vi "Encoder Sim.vi"(2 "Direction":enum16{"A leads B, CCW", "B leads A, CW"}(ring), 3 "Period (s)":dbl=1.0 min=0.001 max=1.0 step=0.001) -> (0 "Actual Counts":i32, 1 "Encoder Signals":bool[](array[boolean]))   [LabVIEW 2017]
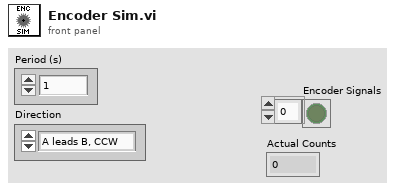
[diagram p1: front panel]
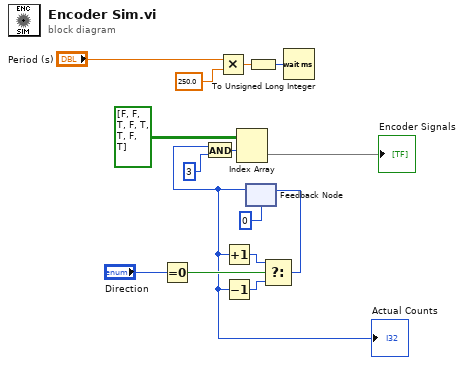
[diagram p0: block diagram]
diagram:
  n1 = Equal To 0?(x="Direction") -> (x = 0?=w8:bool)
  n2 = Multiply(x="Period (s)", y=250.0) -> (x*y=w6:dbl)
  n3 = feedback #1(0) -> (w1:i32)
  "Actual Counts" <- w1
  n4 = And(x=w1, y=3) -> (x .and. y?=w12:i32)
  n5 = Increment(x=w1) -> (x+1=w11:i32)
  n6 = Decrement(x=w1) -> (x-1=w10:i32)
  n7 = Index Array(array=bool[][] [[FALSE, FALSE], [TRUE, FALSE], [TRUE, TRUE], [FALSE, TRUE]], index (row)=w12) -> (element=→"Encoder Signals":bool[])  [unwired: 1 in]
  n8 = To Unsigned Long Integer(number=w6) -> (unsigned 32bit integer=w5:u32)
  n9 = Select(t=w11, s=w8, f=w10) -> (s? t:f=w9:i32)
  n10 = feedback-in #1(w9) -> ()
  n11 = Wait (ms)(milliseconds to wait=w5) -> ()  [unwired: 1 out]
